vi "image labeler.vi"(7 "background opacity":dbl=50.0, 8 "error in (no error)":errorcluster, 9 "[user-specified font]":T3={"Font Name:"="helvetica", "Size"=18, "Strikeout?"=FALSE, "Italic?"=FALSE, "Underline?"=FALSE, "Outline?"=FALSE, "Shadow?"=FALSE, "Bold?"=FALSE}, 10 "text":string, 11 "picture":picture) -> (0 "error out":errorcluster, 3 "new picture":picture)   [LabVIEW 2009]
uses:
  <vilib>/picture/picture.llb/Draw True-Color Pixmap.vi
panel:
  in  "text orientation":T1(ring)
  in  "alignment(left, top)":T2
  in  "origin":cluster{"x":i16, "y":i16}
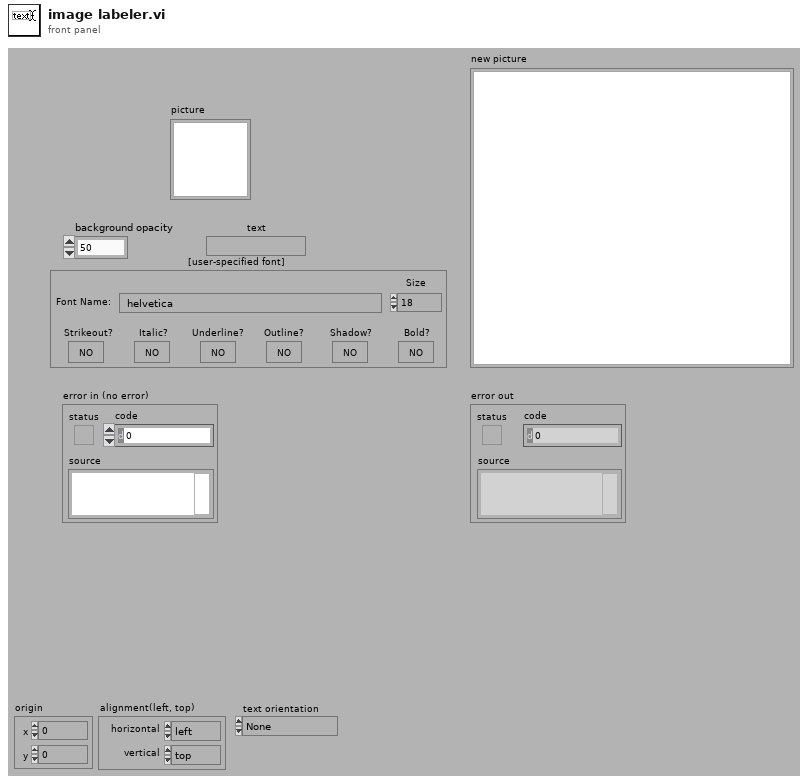
[diagram p1: front panel]
types:
  T1 = enum16{"None", "Stacked", "Clockwise", "Counterclockwise"}
  T2 = cluster{"horizontal":enum16{"left", "center", "right"}, "vertical":enum16{"top", "center", "bottom"}}
  T3 = cluster{"Font Name:":string, "Size":i16, "Strikeout?":bool, "Italic?":bool, "Underline?":bool, "Outline?":bool, "Shadow?":bool, "Bold?":bool}
  T4 = cluster{"y index":i16, "y length":i16, "x index":i16, "x length":i16}
  T5 = enum16{"User-specified Font", "Application Font", "System Font", "Dialog Font"}
  T6 = cluster{"left":i16, "top":i16, "right":i16, "bottom":i16}
  T7 = typedef "imagedata.ctl" = cluster{"image type":i32, "image depth":i32, "image":u8[], "mask":u8[], "colors":u32[], "Rectangle":cluster{"left":i16, "top":i16, "right":i16, "bottom":i16}}
  T8 = cluster{"[user-specified font]":cluster{"Font Name:":string, "Size":i16, "Strikeout?":bool, "Italic?":bool, "Underline?":bool, "Outline?":bool, "Shadow?":bool, "Bold?":bool}, "desired font(Application)":enum16{"User-specified Font", "Application Font", "System Font", "Dialog Font"}, "text orientation ":enum16{"None", "Stacked", "Clockwise", "Counterclockwise"}, "rect":cluster{"left":i16, "top":i16, "right":i16, "bottom":i16}, "text":string}
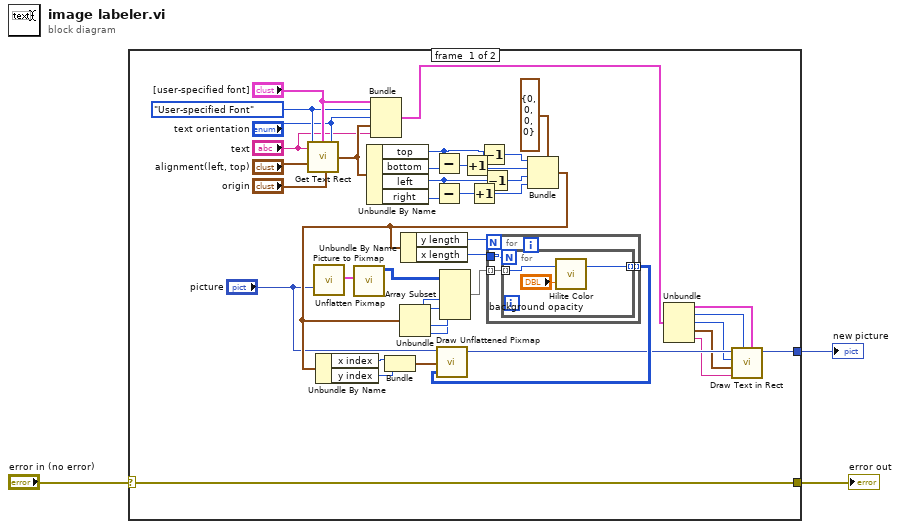
[diagram p0: block diagram]
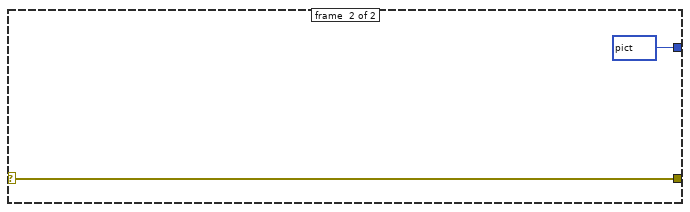
[diagram p2: hidden frame]
diagram:
  n1 = case shown="Error" "error in (no error)" {
    selector: "error in (no error)" -> [w4 w53]
    tunnel: [w45 picture bytes[48] ("new picture")] -> w3
    tunnel: [w4 w53] -> w1
    frame #0 {
      w16 = T5."User-specified Font" ("desired font(Application)")
      n2 = call <vilib>:"Get Text Rect.vi"("alignment(left, top)"="alignment(left, top)", "desired font(Application)"=w16, "origin(0,0)"="origin", "text"="text", "text orientation"="text orientation", "[user-specified font]"="[user-specified font]") -> ("rect"=w14:T6)  [unwired: 3 in]
      n3 = call <vilib>:"Picture to Pixmap.vi"("picture"="picture") -> ("image data"=w42:T7)  [unwired: 9 in, 1 out]
      n4 = call <vilib>:"Unflatten Pixmap.vi"("image data"=w42) -> ("24-bit pixmap"=w24:u32[][])  [unwired: 4 in, 6 out]
      n5 = Unbundle By Name(w14) -> ("top"=w36:i16, "bottom"=w41:i16, "left"=w38:i16, "right"=w40:i16)
      n6 = Bundle("[user-specified font]"="[user-specified font]", "desired font(Application)"=w16, "text orientation"="text orientation", "rect"=w14, "text"="text") -> (w11:T8)  [unwired: 1 in]
      n7 = Subtract(x=w36, y=w41) -> (x-y=w39:i16)
      n8 = Subtract(x=w38, y=w40) -> (x-y=w37:i16)
      n9 = Increment(x=w39) -> (x+1=w34:i16)
      n10 = Increment(x=w37) -> (x+1=w32:i16)
      n11 = Decrement(x=w36) -> (x-1=w35:i16)
      n12 = Decrement(x=w38) -> (x-1=w33:i16)
      n13 = Bundle(cluster=T4 {"y index"=0, "y length"=0, "x index"=0, "x length"=0}, "y index"=w35, "y length"=w34, "x index"=w33, "x length"=w32) -> (w12:T4)
      n14 = Unbundle By Name(w12) -> ("x index"=w22:i16, "y index"=w23:i16)
      n15 = Bundle("x index"=w22, "y index"=w23) -> (w21:cluster{"x index":i16, "y index":i16})  [unwired: 1 in]
      n16 = Unbundle(w12) -> ("y index"=w31:i16, "y length"=w30:i16, "x index"=w29:i16, "x length"=w28:i16)
      n17 = Unbundle By Name(w12) -> ("y length"=w26:i16, "x length"=w25:i16)
      n18 = Array Subset(array=w24, index (row)=w31, length (row)=w30, index (col)=w29, length (col)=w28) -> (w18:u32[][])
      n19 = for {
        N: w26 -> [_]
        tunnel: w25 -> [w48]
        tunnel: w18 -> [w47] mode=indexing
        tunnel: [w46] -> w20 mode=indexing
        n20 = for {
          N: w48 -> [_]
          tunnel: w47 -> [w50] mode=indexing
          tunnel: [w49] -> w46 mode=indexing
          n21 = call <vilib>:"Hilite Color.vi"("Percentage(30)"="background opacity", "Color In"=w50) -> ("Hilite"=w49:u32)  [unwired: 1 out]
        }
      }
      n22 = call-poly <vilib>:"Draw Unflattened Pixmap.vi"("picture"="picture", "top left point(0, 0)"=w21, "data (RGB format)"=w20) -> ("new picture"=w19:picture)  [unwired: 6 in]
      n23 = Unbundle(w11) -> ("[user-specified font]"=w10:T3, "desired font(Application)"=w9:T5, "text orientation"=w8:T1, "rect"=w7:T6, "text"=w6:string)
      n24 = call <vilib>:"Draw Text in Rect.vi"("[user-specified font]"=w10, "desired font(Application)"=w9, "text"=w6, "rect"=w7, "text orientation"=w8, "picture"=w19) -> ("new picture"=w45:picture)  [unwired: 5 in]
    }
    frame #1 {
    }
  }
  "new picture" <- w3
  "error out" <- w1
